vi "Delete last data.vi"(8 "error in (no error)":errorcluster, 11 "Directory":string[](array[string])) -> (0 "error out":errorcluster)   [LabVIEW 2017]
uses:
  Control/Folder Format.ctl
  File.lvlib
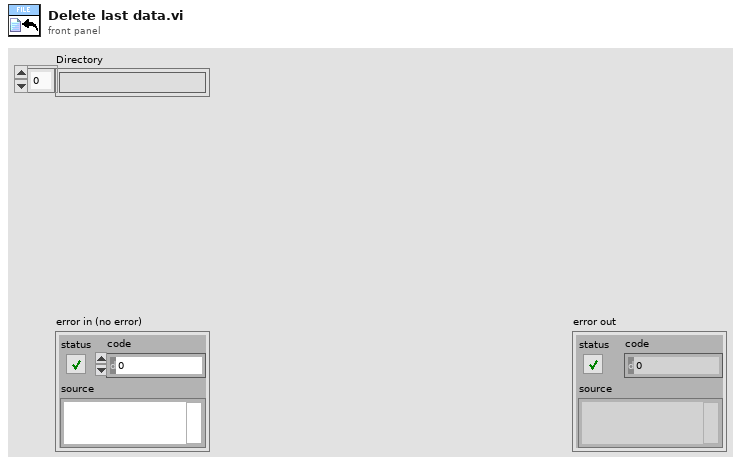
[diagram p1: front panel]
types:
  T1 = typedef "File.lvlib/Folder Format.ctl" = enum16{"None", "Folder Date", "Folder/Date"}
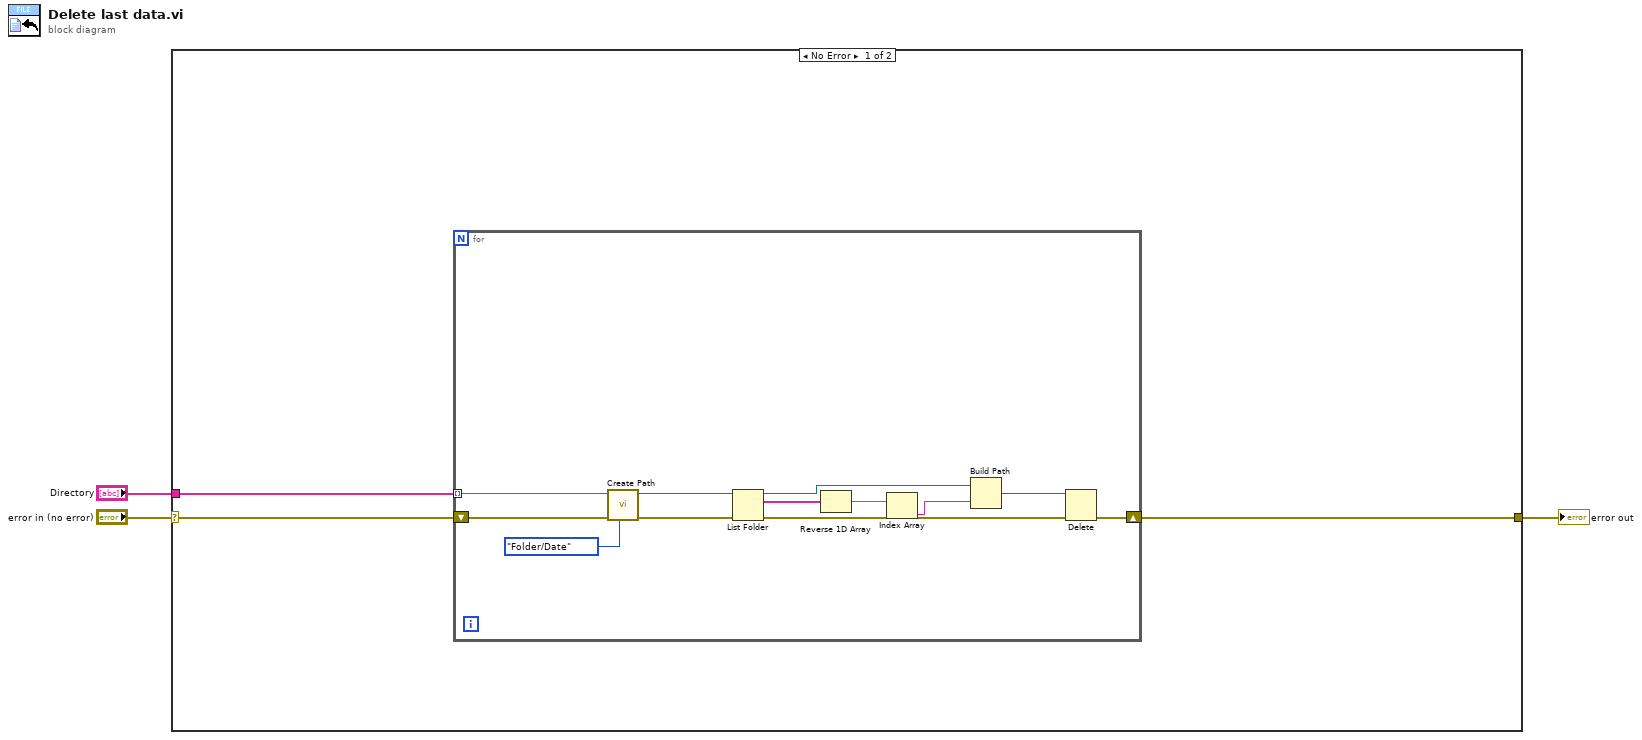
[diagram p0: block diagram]
diagram:
  n1 = case shown="No Error" "error in (no error)" {
    selector: "error in (no error)" -> [w6 w19]
    tunnel: [w5 w19] -> w2
    tunnel: "Directory" -> [w4 _]
    frame No Error {
      n2 = for {
        shift-right: [w9] -> w5
        shift-left: w6 -> [w18]
        tunnel: w4 -> [w7] mode=indexing
        n3 = call "Create Path.vi"("Folder Format"=Folder_Format."Folder/Date", "error in (no error)"=w18, "Directory"=w7) -> ("error out"=w17:errorcluster, "Path"=w16:path)  [unwired: 7 in]
        n4 = List Folder(path=w16, error in=w17) -> (path out=w13:path, filenames=w15:string[], error out=w11:errorcluster)  [unwired: 2 in, 1 out]
        n5 = Reverse 1D Array(array=w15) -> (reversed array=w14:string[])
        n6 = Index Array(array=w14) -> (element=w12:string)  [unwired: 1 in]
        n7 = Build Path(base path=w13, name or relative path=w12) -> (appended path=w10:path)
        n8 = Delete(path (use dialog)=w10, error in=w11) -> (error out=w9:errorcluster)  [unwired: 3 in, 2 out]
      }
    }
    frame Error {
    }
  }
  "error out" <- w2
